vi "Demo VI.vi"() -> ()   [LabVIEW 2016]
panel:
  out "VI Name":string
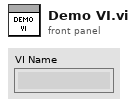
[diagram p1: front panel]
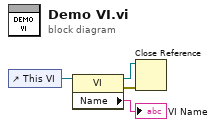
[diagram p0: block diagram]
diagram:
  n1 = control-ref of="This VI"() -> (w4:refnum<vi>)
  n2 = property class="VI"(reference=w4) -> (reference out=w1:refnum<vi>, error out=w2:errorcluster, "Name"=→"VI Name":string)  [unwired: 1 in]
  n3 = Close Reference(reference=w1, error in (no error)=w2) -> ()  [unwired: 1 out]
